vi "LEP_RV_OpBox.vi"() -> (11 "Text":string=".")   [LabVIEW 2011]
uses:
  LEP_RV_OpBoxGlobal.vi
panel:
  in  "stop":bool caption="Stop"
  out "Text 2":string="Initializing operation."
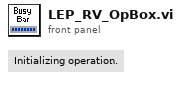
[diagram p1: front panel]
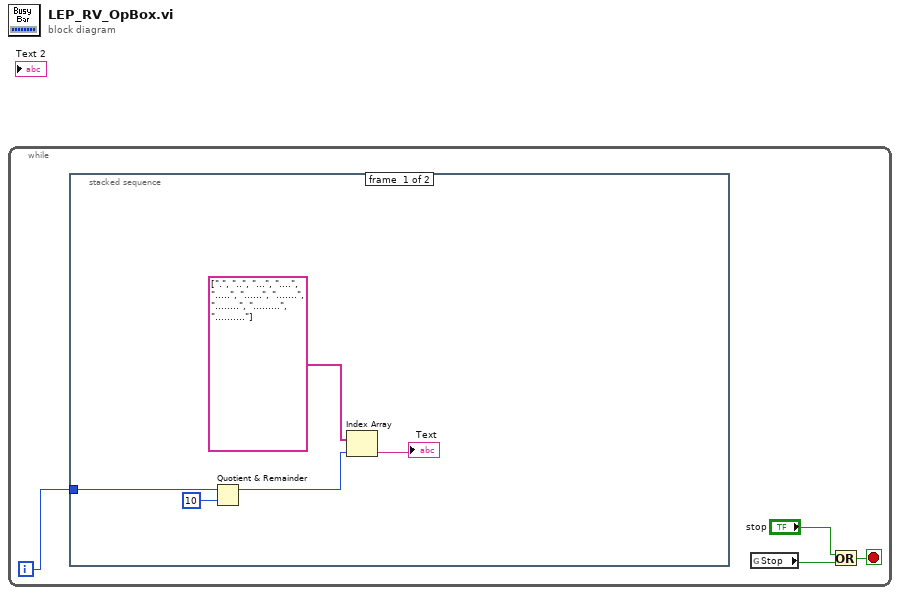
[diagram p0: block diagram]
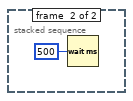
[diagram p2: hidden frame]
diagram:
  n1 = while {
    i -> [w4]
    stop <- w3 stop-if-true
    n2 = stacked-sequence {
      tunnel: w4 -> [w9 _]
      frame #0 {
        n3 = Quotient & Remainder(x=w9, y=10) -> (x-y*floor(x/y)=w6:i32)  [unwired: 1 out]
        n4 = Index Array(array=string[] [".", "..", "...", "....", ".....", "......", ".......", "........", ".........", ".........."], index=w6) -> (element=→"Text":string)
      }
      frame #1 {
        n5 = Wait (ms)(milliseconds to wait=u32 500) -> ()  [unwired: 1 out]
      }
    }
    n6 = global read "LEP_RV_OpBoxGlobal.vi" "Stop"() -> (w1:bool)
    n7 = Or(x="stop", y=w1) -> (x .or. y?=w3:bool)
  }
